vi "client.vi"() -> ()   [LabVIEW 2018]
panel:
  in  "设备信息":T1
  in  "停止":bool
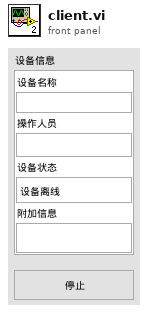
[diagram p1: front panel]
types:
  T1 = cluster{"设备名称":string, "操作人员":string, "设备状态":enum16{"设备离线", "设备正常", "设备缺料", "设备故障", "质量报警"}, "附加信息":string}
  T2 = cluster{"设备名称":bool, "操作人员":bool, "设备状态":bool, "附加信息":bool}
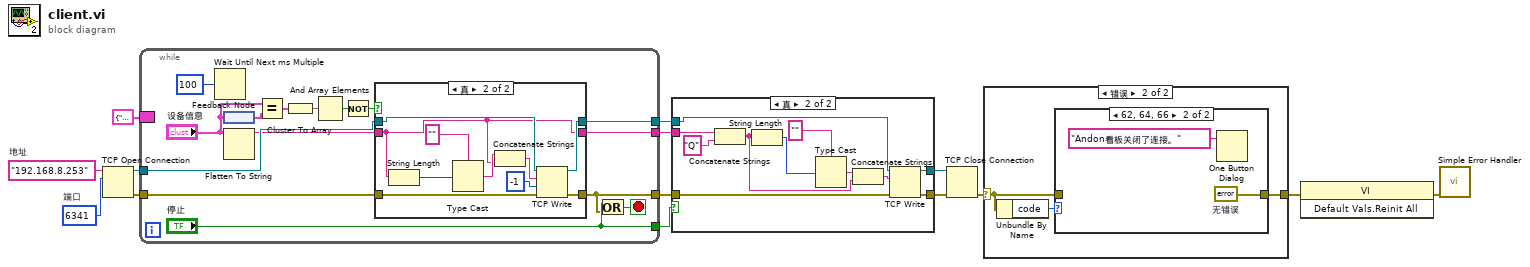
[diagram p0: block diagram]
diagram:
  w13 = u16 6341  # 端口
  w14 = "192.168.8.253"  # 地址
  n1 = TCP Open Connection(address=w14, remote port or service name=w13) -> (connection ID=w12:refnum<k5>, error out=w11:errorcluster)  [unwired: 1 in, 2 out]
  n2 = while {
    tunnel: ["停止"] -> w6
    tunnel: [w27] -> w10
    tunnel: [w24] -> w8
    tunnel: w11 -> [w28]
    tunnel: w12 -> [w29]
    tunnel: [w17] -> w4
    border: T1 {"设备名称"="", "操作人员"="", "设备状态"=enum."设备正常", "附加信息"=""} ("设备信息") -> [_]
    stop <- w26 stop-if-true
    n3 = Wait Until Next ms Multiple(millisecond multiple=u32 100 ("毫秒倍数")) -> ()  [unwired: 1 out]
    n4 = feedback-in #1("设备信息") -> ()
    n5 = feedback #1() -> (w21:T1)
    n6 = Flatten To String(anything="设备信息") -> (data string=w18:string)  [unwired: 3 in, 2 out]
    n7 = Equal?(x="设备信息", y=w21) -> (x = y?=w20:T2)
    n8 = Cluster To Array(cluster=w20) -> (array=w19:bool[])
    n9 = And Array Elements(Boolean array=w19) -> (logical AND=w16:bool)
    n10 = Not(x=w16) -> (.not. x?=w15:bool)
    n11 = case shown="真" w15 {
      tunnel: w29 -> [w32 w42]
      tunnel: w28 -> [w31 w41]
      tunnel: [w32 w40] -> w27
      tunnel: [w31 w39] -> w24
      tunnel: w18 -> [w30 w33]
      tunnel: [w30 w33] -> w17
      frame False {
      }
      frame True {
        n12 = String Length(string=w33) -> (length=w37:i32)
        n13 = Type Cast(type="", x=w37) -> (*(type *) &x=w35:string)
        n14 = Concatenate Strings(w35, w33) -> (w34:string)
        n15 = TCP Write(connection ID=w42, data in=w34, error in (no error)=w41, 9:-1) -> (connection ID out=w40:refnum<k5>, error out=w39:errorcluster)  [unwired: 1 out]
      }
    }
    n16 = Or(x="停止", y=w24) -> (x .or. y?=w26:bool)
  }
  n17 = case shown="真" w6 {
    tunnel: w10 -> [w44 w55]
    tunnel: [w44 w53] -> w9
    tunnel: w8 -> [w43 w54]
    tunnel: [w43 w52] -> w7
    tunnel: w4 -> [_ w50]
    frame False {
    }
    frame True {
      n18 = Concatenate Strings(w50, "Q") -> (w46:string)
      n19 = String Length(string=w46) -> (length=w49:i32)
      n20 = Type Cast(type="", x=w49) -> (*(type *) &x=w47:string)
      n21 = Concatenate Strings(w47, w46) -> (w45:string)
      n22 = TCP Write(connection ID=w55, data in=w45, error in (no error)=w54) -> (connection ID out=w53:refnum<k5>, error out=w52:errorcluster)  [unwired: 2 out]
    }
  }
  n23 = TCP Close Connection(connection ID=w9, error in (no error)=w7) -> (error out=w5:errorcluster)  [unwired: 2 out]
  n24 = case shown="错误" w5 {
    selector: w5 -> [w56 w58]
    tunnel: [w56 w57] -> w2
    frame No Error {
    }
    frame Error {
      n25 = Unbundle By Name(w58) -> ("code"=w59:i32)
      n26 = case shown="62, 64, 66" w59 {
        tunnel: w58 -> [w60 _]
        tunnel: [w60 w62] -> w57
        frame Default {
        }
        frame 62, 64, 66 {
          w62 = errorcluster {"status"=FALSE, "code"=0, "source"=""}  # 无错误
          n27 = One Button Dialog(message="Andon看板关闭了连接。" ("服务器关闭")) -> ()  [unwired: 1 in, 1 out]
        }
      }
    }
  }
  n28 = invoke class="VI" method="Default Vals.Reinit All"(error in=w2) -> (error out=w1:errorcluster)  [unwired: 2 in, 2 out]
  n29 = call <vilib>:"Simple Error Handler.vi"("error in (no error)"=w1) -> ()  [unwired: 1 in, 8 out]
